vi "Initalize.vi"(8 "error in (no error)":errorcluster, 9 "Path":path, 10 "Section":string, 11 "Sim Laser Driver in":refnum<class "Sim Laser Driver.lvclass">) -> (0 "error out":errorcluster, 3 "Sim Laser Driver out":refnum<class "Sim Laser Driver.lvclass">)   [LabVIEW 2022 SP3, in "Sim Laser Driver.lvclass"]
uses:
  Sim Laser Driver.lvclass
  C:/XY Stage/XY Stage/Framework/Base/Base.lvclass
  data.ctl
  settings.ctl
  XY Stage/Framework/Base/Base.lvclass/Base.ctl
  Sim Laser Driver.lvclass/Sim Laser Driver.ctl
  XY Stage/Framework/Base/Accessors/Write Config Path.vi
  XY Stage/Framework/Base/Accessors/Write Section.vi
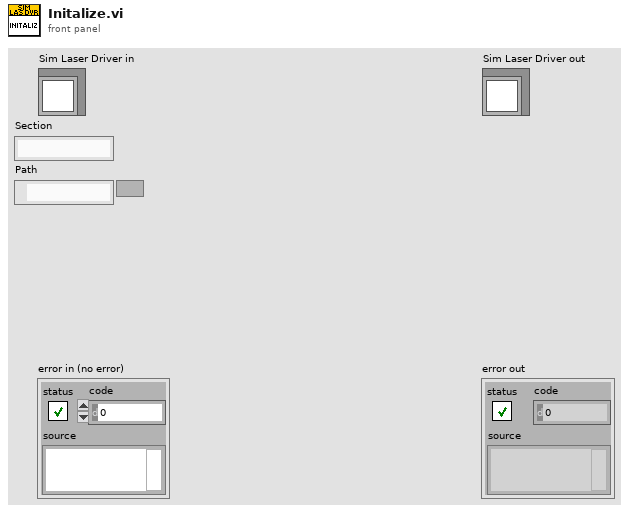
[diagram p1: front panel]
types:
  T1 = typedef "Sim Laser Driver.lvclass/data.ctl" = cluster{"Settings":T2, "Warming":bool, "Firing":bool, "Current Temp":dbl}
  T2 = typedef "Sim Laser Driver.lvclass/settings.ctl" = cluster{"Power":dbl}
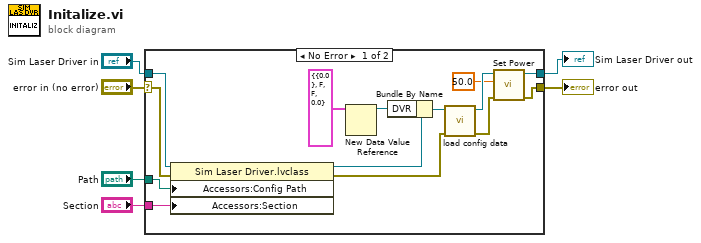
[diagram p0: block diagram]
diagram:
  n1 = case shown="No Error" "error in (no error)" {
    selector: "error in (no error)" -> [w16 w22]
    tunnel: [w7 w22] -> w5
    tunnel: [w9 w21] -> w3
    tunnel: "Sim Laser Driver in" -> [w20 w21]
    tunnel: "Path" -> [w19 _]
    tunnel: "Section" -> [w18 _]
    frame No Error {
      n2 = property class="Sim Laser Driver.lvclass"(reference=w20, error in=w16, "Accessors:Config Path"=w19, "Accessors:Section"=w18) -> (reference out=w17:refnum<class "Sim Laser Driver.lvclass">, error out=w15:errorcluster)
      n3 = New Data Value Reference(data value=T1 {"Settings"={"Power"=0.0}, "Warming"=FALSE, "Firing"=FALSE, "Current Temp"=0.0} ("data")) -> (data value reference=w12:refnum<data-value>)  [unwired: 1 in, 1 out]
      n4 = Bundle By Name(cluster=w17, "DVR"=w12) -> (w13:refnum<class "Sim Laser Driver.lvclass">)
      n5 = call-dynamic "load config data.vi"("error in (no error)"=w15, "Sim Laser Driver in"=w13) -> ("error out"=w8:errorcluster, "Sim Laser Driver out"=w11:refnum<class "Sim Laser Driver.lvclass">)  [unwired: 8 in]
      n6 = call-dynamic "Set Power.vi"("error in (no error)"=w8, "Power Percentage"=50.0, "Sim Laser Driver in"=w11) -> ("error out"=w7:errorcluster, "Sim Laser Driver out"=w9:refnum<class "Sim Laser Driver.lvclass">)  [unwired: 7 in]
    }
    frame Error {
    }
  }
  "error out" <- w5
  "Sim Laser Driver out" <- w3
